vi "Lookup Reference FGV.vi"(7 "State":T2, 8 "error in":errorcluster, 9 "index":i32, 10 "Query ref in":T1, 11 "VISA In":refnum<visa-resource-name>) -> (0 "error out":errorcluster, 1 "Found Ref?":bool, 2 "Query ref":T1, 3 "VISA Out":refnum<visa-resource-name>)   [LabVIEW 2014, in "Mercury iXX.lvlib"]
uses:
  Mercury iXX.lvlib
  Controls/Lookup Reference FGV Enum.ctl
  Controls/Query Dynamic Reference.ctl
  Controls/VI Ref Lookup Cluster.ctl
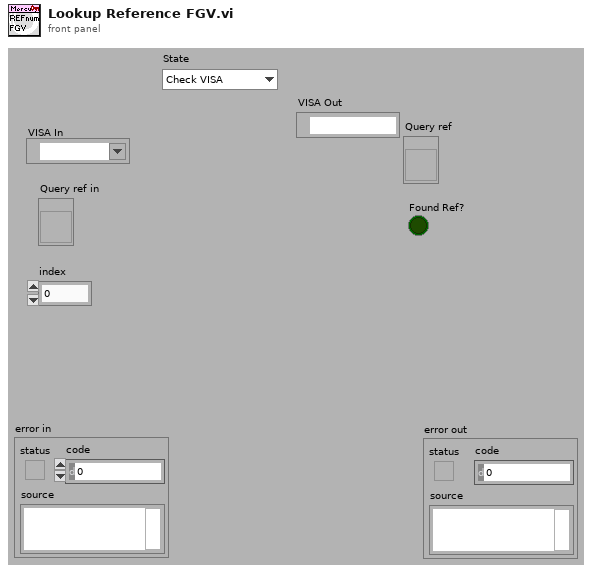
[diagram p1: front panel]
types:
  T1 = typedef "Mercury iXX.lvlib/Query Dynamic Reference.ctl" = refnum<vi>
  T2 = typedef "Mercury iXX.lvlib/Lookup Reference FGV Enum.ctl" = enum16{"Check VISA", "Get VI Ref", "Set VI ref", "Delete Single Ref", "Clear All"}
  T3 = typedef "Mercury iXX.lvlib/VI Ref Lookup Cluster.ctl" = cluster{"Visa Ref Array":refnum<visa-resource-name>[], "VI Ref Array":T1[]}
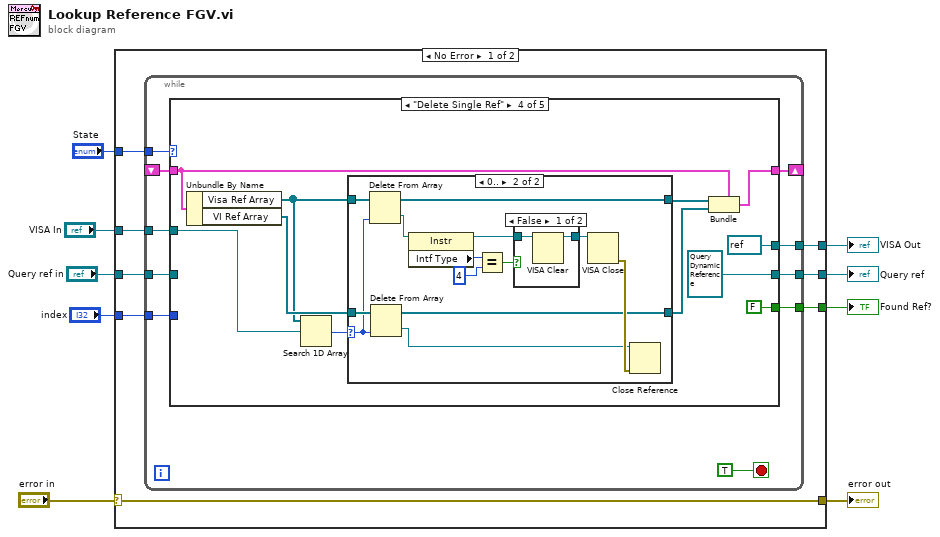
[diagram p0: block diagram]
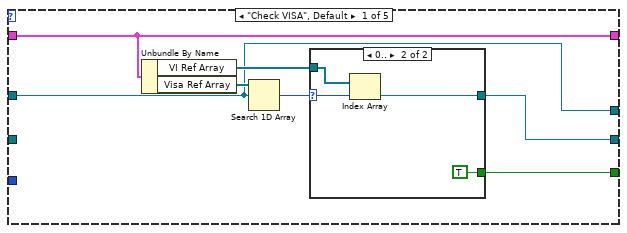
[diagram p2: hidden frame]
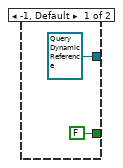
[diagram p3: hidden frame]
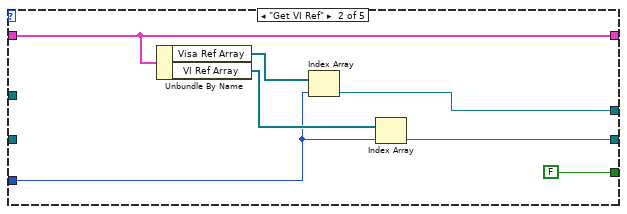
[diagram p4: hidden frame]
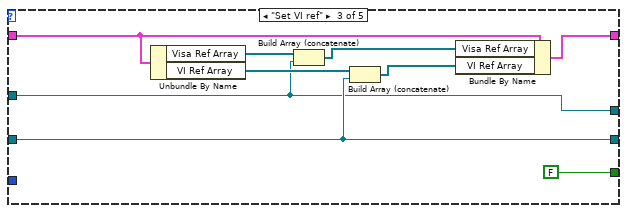
[diagram p5: hidden frame]
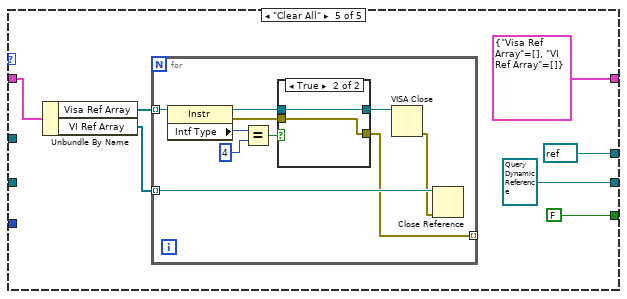
[diagram p8: hidden frame]
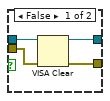
[diagram p9: hidden frame]
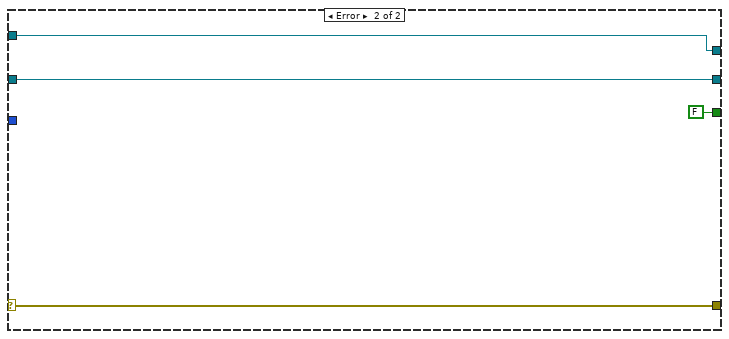
[diagram p10: hidden frame]
diagram:
  n1 = case shown="No Error" "error in" {
    selector: "error in" -> [w10 w112]
    tunnel: "State" -> [w17 _]
    tunnel: "VISA In" -> [w16 w111]
    tunnel: [w15 FALSE] -> w7
    tunnel: [w14 w110] -> w6
    tunnel: "Query ref in" -> [w13 w110]
    tunnel: "index" -> [w12 _]
    tunnel: [w11 w111] -> w3
    tunnel: [w10 w112] -> w1
    frame No Error {
      n2 = while {
        shift-right: [w27] -> _
        shift-left: _ -> [w24]
        tunnel: w17 -> [w25]
        tunnel: w16 -> [w23]
        tunnel: [w22] -> w15
        tunnel: [w21] -> w14
        tunnel: w13 -> [w20]
        tunnel: w12 -> [w19]
        tunnel: [w18] -> w11
        stop <- TRUE stop-if-true
        n3 = case shown="\"Delete Single Ref\"" w25 {
          tunnel: [w30 w47 w55 w59 T3 {"Visa Ref Array"=[], "VI Ref Array"=[]} ("VI Ref Lookup Cluster")] -> w27
          tunnel: w24 -> [w30 w47 w56 w60 w88]
          tunnel: w23 -> [w28 _ w48 w62 _]
          tunnel: [w32 FALSE FALSE FALSE FALSE] -> w22
          tunnel: [w29 w43 w50 T1 refnum ("Query ref in") T1 refnum ("Query ref in")] -> w21
          tunnel: w20 -> [_ _ w50 _ _]
          tunnel: w19 -> [_ w44 _ _ _]
          tunnel: [w28 w42 w48 refnum<visa-resource-name> refnum ("VISA In") refnum<visa-resource-name> refnum ("VISA In")] -> w18
          frame "Check VISA", Default {
            n4 = Unbundle By Name(w30) -> ("VI Ref Array"=w31:T1[], "Visa Ref Array"=w34:refnum<visa-resource-name>[])
            n5 = Search 1D Array(1D array=w34, element=w28) -> (index of element=w33:i32)  [unwired: 1 out]
            n6 = case shown="0.." w33 {
              selector: w33 -> [_ w38]
              tunnel: [FALSE TRUE] -> w32
              tunnel: w31 -> [_ w39]
              tunnel: [T1 refnum ("Query reference") w37] -> w29
              frame -1, Default {
              }
              frame 0.. {
                n7 = Index Array(array=w39, index=w38) -> (element=w37:T1)
              }
            }
          }
          frame "Get VI Ref" {
            n8 = Unbundle By Name(w47) -> ("Visa Ref Array"=w46:refnum<visa-resource-name>[], "VI Ref Array"=w45:T1[])
            n9 = Index Array(array=w46, index=w44) -> (element=w42:refnum<visa-resource-name>)
            n10 = Index Array(array=w45, index=w44) -> (element=w43:T1)
          }
          frame "Set VI ref" {
            n11 = Unbundle By Name(w56) -> ("Visa Ref Array"=w54:refnum<visa-resource-name>[], "VI Ref Array"=w53:T1[])
            n12 = Build Array (concatenate)(w54, w48) -> (w52:refnum<visa-resource-name>[])
            n13 = Build Array (concatenate)(w53, w50) -> (w51:T1[])
            n14 = Bundle By Name(cluster=w56, "Visa Ref Array"=w52, "VI Ref Array"=w51) -> (w55:T3)
          }
          frame "Delete Single Ref" {
            n15 = Unbundle By Name(w60) -> ("Visa Ref Array"=w63:refnum<visa-resource-name>[], "VI Ref Array"=w64:T1[])
            n16 = Search 1D Array(1D array=w63, element=w62) -> (index of element=w61:i32)  [unwired: 1 out]
            n17 = case shown="0.." w61 {
              selector: w61 -> [_ w77]
              tunnel: w64 -> [w68 w80]
              tunnel: w63 -> [w69 w78]
              tunnel: [w69 w76] -> w58
              tunnel: [w68 w75] -> w57
              frame -1, Default {
              }
              frame 0.. {
                n18 = Delete From Array(array=w78, index=w77) -> (deleted portion=w74:refnum<visa-resource-name>, array with subset deleted=w76:refnum<visa-resource-name>[])  [unwired: 1 in]
                n19 = Delete From Array(array=w80, index=w77) -> (deleted portion=w79:T1, array with subset deleted=w75:T1[])  [unwired: 1 in]
                n20 = property class="Instr"(reference=w74) -> (reference out=w73:refnum<visa-resource-name>, "Intf Type"=w72:u16)  [unwired: 1 in, 1 out]
                n21 = Equal?(x=w72, y=u16 4) -> (x = y?=w70:bool)
                n22 = case shown="False" w70 {
                  tunnel: [w84 w85] -> w82
                  tunnel: w73 -> [w83 w85]
                  frame False {
                    n23 = VISA Clear(VISA resource name=w83) -> (VISA resource name out=w84:refnum<visa-resource-name>)  [unwired: 1 in, 1 out]
                  }
                  frame True {
                  }
                }
                n24 = VISA Close(VISA resource name=w82) -> (error out=w81:errorcluster)  [unwired: 1 in]
                n25 = Close Reference(reference=w79, error in (no error)=w81) -> ()  [unwired: 1 out]
              }
            }
            n26 = Bundle(cluster=w60, "Visa Ref Array"=w58, "VI Ref Array"=w57) -> (w59:T3)
          }
          frame "Clear All" {
            n27 = Unbundle By Name(w88) -> ("Visa Ref Array"=w87:refnum<visa-resource-name>[], "VI Ref Array"=w86:T1[])
            n28 = for {
              tunnel: w87 -> [w98] mode=indexing
              tunnel: w86 -> [w101] mode=indexing
              tunnel: [w99] -> _ mode=indexing
              n29 = property class="Instr"(reference=w98) -> (reference out=w93:refnum<visa-resource-name>, error out=w94:errorcluster, "Intf Type"=w97:u16)  [unwired: 1 in]
              n30 = Equal?(x=w97, y=u16 4) -> (x = y?=w95:bool)
              n31 = case shown="True" w95 {
                tunnel: [w106 w108] -> w102
                tunnel: [w105 w107] -> w99
                tunnel: w94 -> [w104 w107]
                tunnel: w93 -> [w103 w108]
                frame False {
                  n32 = VISA Clear(VISA resource name=w103, error in (no error)=w104) -> (VISA resource name out=w106:refnum<visa-resource-name>, error out=w105:errorcluster)
                }
                frame True {
                }
              }
              n33 = VISA Close(VISA resource name=w102) -> (error out=w100:errorcluster)  [unwired: 1 in]
              n34 = Close Reference(reference=w101, error in (no error)=w100) -> ()  [unwired: 1 out]
            }
          }
        }
      }
    }
    frame Error {
    }
  }
  "error out" <- w1
  "Found Ref?" <- w7
  "Query ref" <- w6
  "VISA Out" <- w3
